vi "Drive and Climb SS Implem 2017.vi"(11 "Robot Commands":T2) -> (3 "Drive Actuator Out":T1={"Left Drive Output"=0.0, "Right Drive Output"=0.0, "Low/High Gear Shift"=enum."Reverse", "Left Climb Shift"=enum."Off", "Right Climb Shift"=enum."Off", "Run Climb Motor"=0.0})   [LabVIEW 2016]
uses:
  Drive + Climb Commands 2017.ctl
  Drive Actuator Out 2017.ctl
  Global Variables/Robot Status.vi
  Global Variables/High Gear Calibrations.vi
  Global Variables/Low Gear Calibrations.vi
  Global Variables/Auto Drive Calibrations.vi
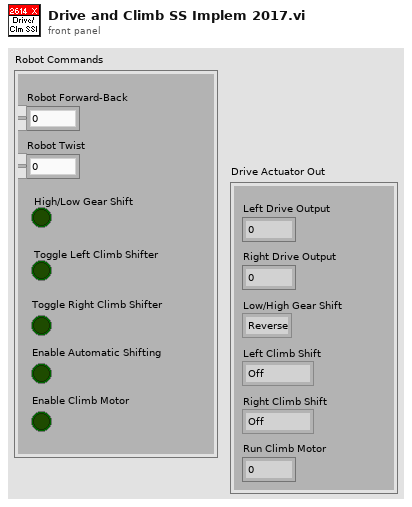
[diagram p1: front panel]
types:
  T1 = typedef "Drive Actuator Out 2017.ctl" = cluster{"Left Drive Output":dbl, "Right Drive Output":dbl, "Low/High Gear Shift":enum16{"Off", "On", "Forward", "Reverse"}, "Left Climb Shift":enum16{"Off", "On", "Forward", "Reverse"}, "Right Climb Shift":enum16{"Off", "On", "Forward", "Reverse"}, "Run Climb Motor":dbl}
  T2 = typedef "Drive + Climb Commands 2017.ctl" = cluster{"Robot Forward-Back":dbl, "Robot Twist":dbl, "High/Low Gear Shift":bool, "Toggle Left Climb Shifter":bool, "Toggle Right Climb Shifter":bool, "Enable Automatic Shifting":bool, "Enable Climb Motor ":bool}
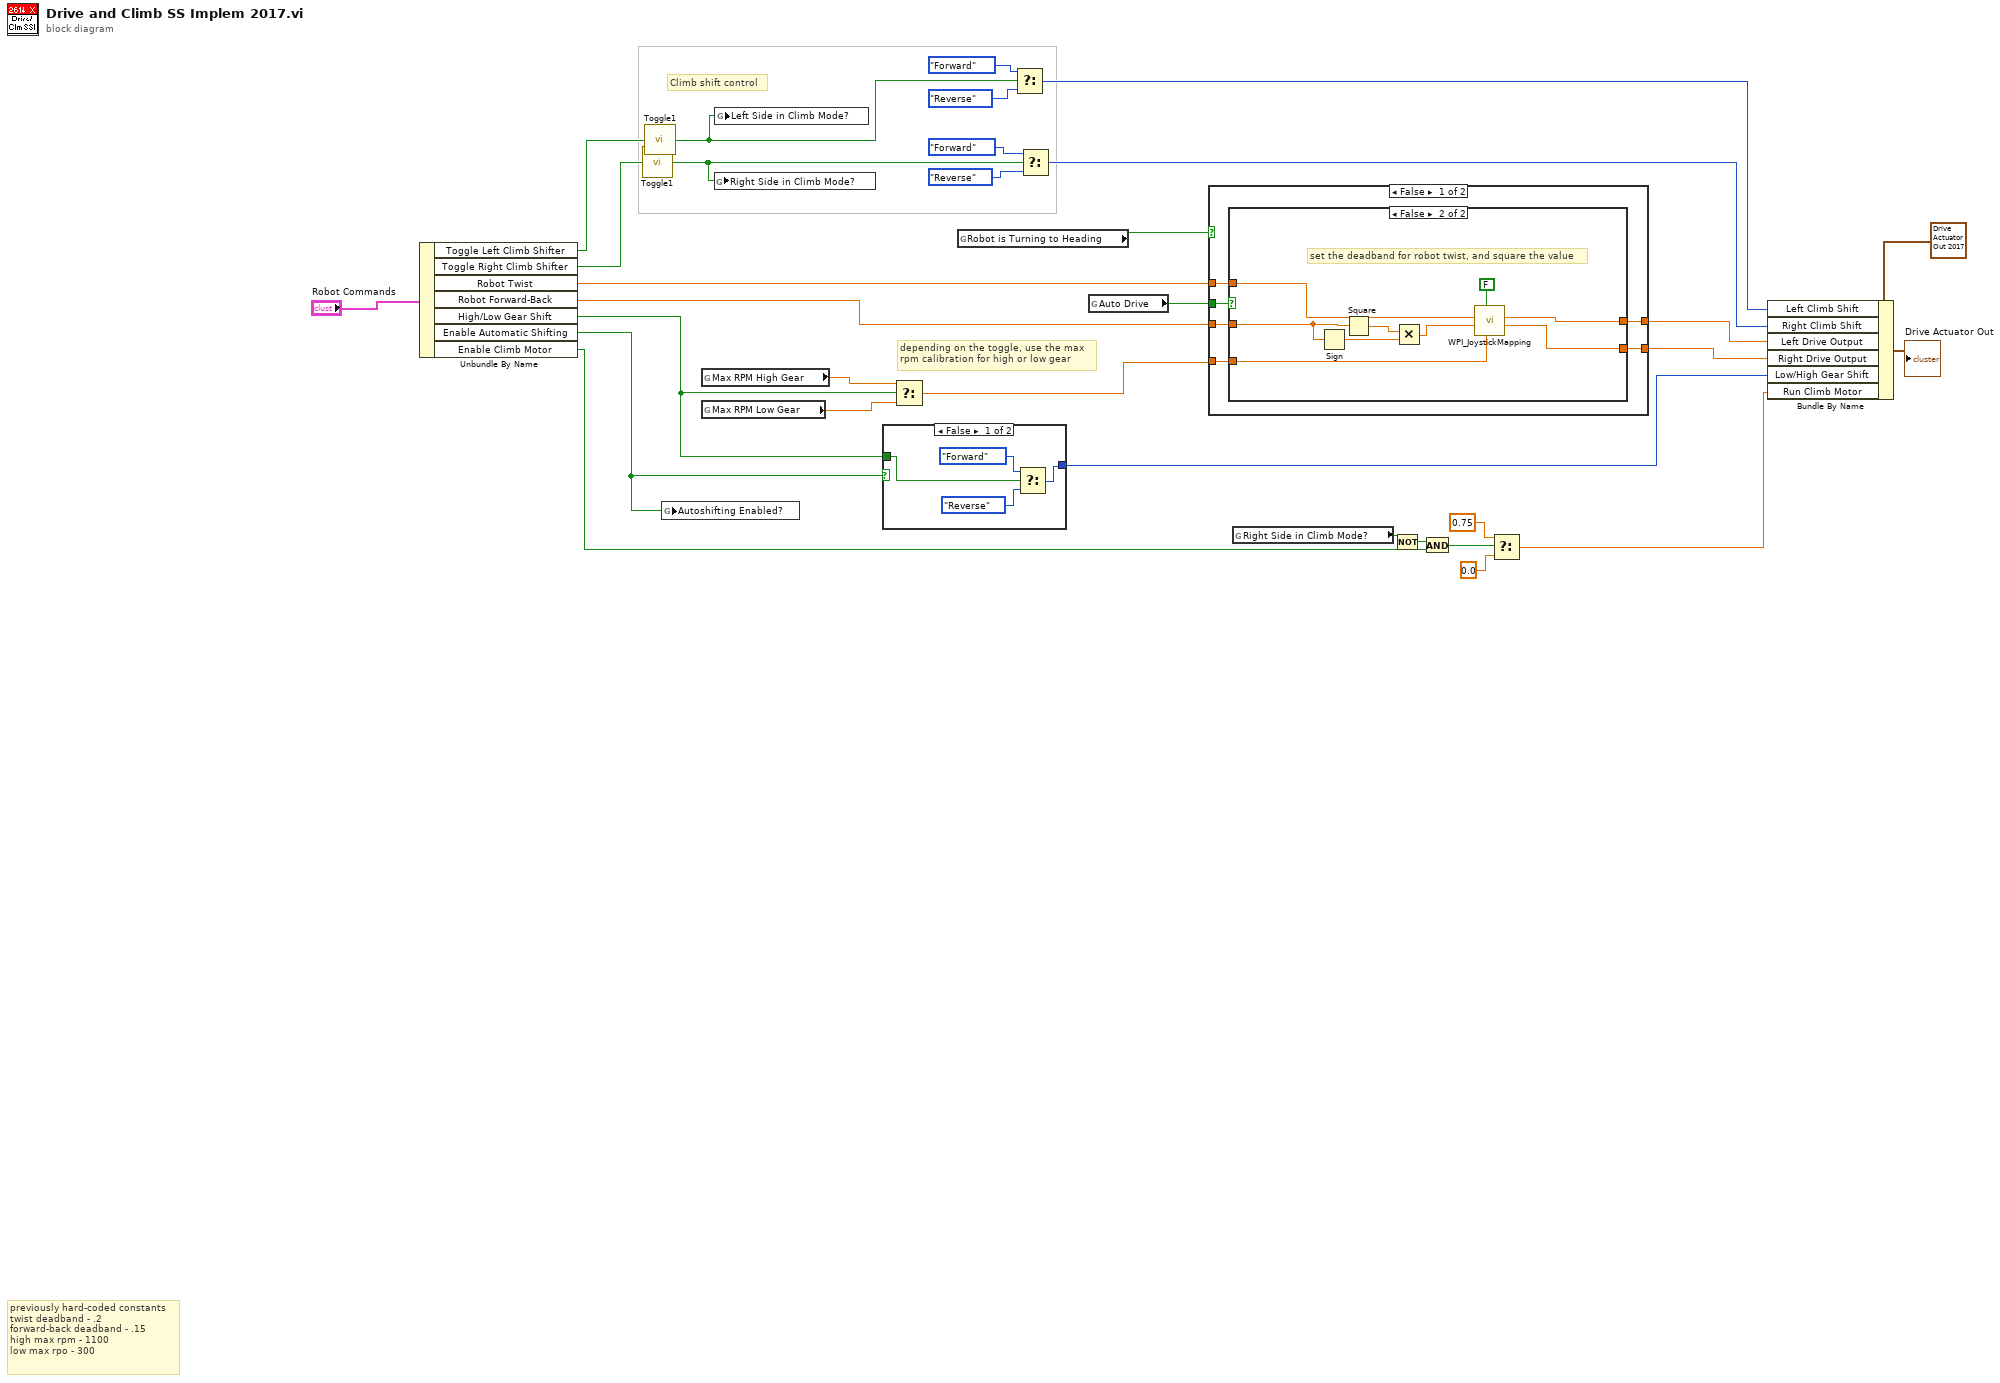
[diagram p0: block diagram]
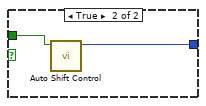
[diagram p2: hidden frame]
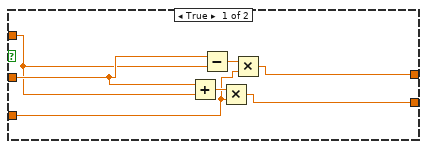
[diagram p3: hidden frame]
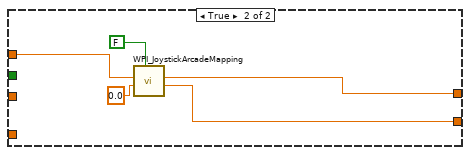
[diagram p4: hidden frame]
diagram:
  # "Climb shift control"
  # "depending on the toggle, use the max\nrpm calibration for high or low gear"
  # "previously hard-coded constants\ntwist deadband - .2\nforward-back deadband - .15\nhigh max rpm - 1100\nlow max rpo - 300"
  n1 = Unbundle By Name("Robot Commands") -> ("Toggle Left Climb Shifter"=w25:bool, "Toggle Right Climb Shifter"=w24:bool, "Robot Twist"=w15:dbl, "Robot Forward-Back"=w10:dbl, "High/Low Gear Shift"=w9:bool, "Enable Automatic Shifting"=w13:bool, "Enable Climb Motor"=w3:bool)
  n2 = call "Toggle1.vi"("Boolean"=w24) -> ("Driver Switch 2"=w16:bool)
  n3 = call "Toggle1.vi"("Boolean"=w25) -> ("Driver Switch 2"=w17:bool)
  n4 = global write "Robot Status.vi" "Autoshifting Enabled?"(w13) -> ()
  n5 = global read "High Gear Calibrations.vi" "Max RPM High Gear"() -> (w26:dbl)
  n6 = global read "Low Gear Calibrations.vi" "Max RPM Low Gear"() -> (w11:dbl)
  n7 = global write "Robot Status.vi" "Right Side in Climb Mode?"(w16) -> ()
  n8 = global write "Robot Status.vi" "Left Side in Climb Mode?"(w17) -> ()
  n9 = case shown="False" w13 {
    tunnel: [w33 w38] -> w12
    tunnel: w9 -> [w35 w37]
    frame False {
      n10 = Select(t=enum16{"Off", "On", "Forward", "Reverse"}."Forward" ("Low/High Gear Shift"), s=w35, f=enum16{"Off", "On", "Forward", "Reverse"}."Reverse" ("Low/High Gear Shift")) -> (s? t:f=w33:enum16{"Off", "On", "Forward", "Reverse"})
    }
    frame True {
      n11 = call "Auto Shift Control.vi"("High/Low Gear Shift"=w37) -> ("Low/High Gear Shift"=w38:enum16{"Off", "On", "Forward", "Reverse"})  [unwired: 10 in]
    }
  }
  n12 = Select(t=w26, s=w9, f=w11) -> (s? t:f=w27:dbl)
  n13 = global read "Robot Status.vi" "Robot is Turning to Heading"() -> (w14:bool)
  n14 = Select(t=enum16{"Off", "On", "Forward", "Reverse"}."Forward" ("Left Climb Shift"), s=w17, f=enum16{"Off", "On", "Forward", "Reverse"}."Reverse" ("Left Climb Shift")) -> (s? t:f=w19:enum16{"Off", "On", "Forward", "Reverse"})
  n15 = Select(t=enum16{"Off", "On", "Forward", "Reverse"}."Forward" ("Left Climb Shift"), s=w16, f=enum16{"Off", "On", "Forward", "Reverse"}."Reverse" ("Left Climb Shift")) -> (s? t:f=w18:enum16{"Off", "On", "Forward", "Reverse"})
  n16 = global read "Auto Drive Calibrations.vi" "Auto Drive"() -> (w8:bool)
  n17 = case shown="False" w14 {
    tunnel: [w42 w63] -> w29
    tunnel: [w43 w62] -> w28
    tunnel: w10 -> [w40 _]
    tunnel: w27 -> [w44 _]
    tunnel: w15 -> [w41 w61]
    tunnel: w8 -> [w39 _]
    frame False {
      n18 = case shown="False" w39 {
        tunnel: w44 -> [w45 w52]
        tunnel: [w50 w59] -> w43
        tunnel: [w51 w58] -> w42
        tunnel: w41 -> [w48 w57]
        tunnel: w40 -> [w49 w56]
        frame True {
          n19 = Add(x=w49, y=w48) -> (x+y=w47:dbl)
          n20 = Subtract(x=w49, y=w48) -> (x-y=w46:dbl)
          n21 = Multiply(x=w47, y=w45) -> (x*y=w50:dbl)
          n22 = Multiply(x=w46, y=w45) -> (x*y=w51:dbl)
        }
        frame False {
          # "set the deadband for robot twist, and square the value"
          n23 = Sign(1:w56) -> (0:w54:dbl)
          n24 = Square(x=w56) -> (x^2=w55:dbl)
          n25 = Multiply(x=w55, y=w54) -> (x*y=w53:dbl)
          n26 = call-poly <vilib>:"WPI_JoystickMapping.vi"("Max Output"=w52, "Square Inputs"=FALSE, "Y axis value"=w53, "X axis value"=w57) -> ("Right Motor Value"=w59:dbl, "Left Motor Value"=w58:dbl)  [unwired: 6 in]
        }
      }
    }
    frame True {
      n27 = call <vilib>:"WPI_JoystickArcadeMapping.vi"("Square Inputs"=FALSE, "Y axis value"=0.0, "X axis value"=w61) -> ("Right Motor Value"=w62:dbl, "Left Motor Value"=w63:dbl)  [unwired: 7 in]
    }
  }
  n28 = global read "Robot Status.vi" "Right Side in Climb Mode?"() -> (w2:bool)
  n29 = Not(x=w2) -> (.not. x?=w1:bool)
  n30 = And(x=w1, y=w3) -> (x .and. y?=w4:bool)
  n31 = Select(t=0.75, s=w4, f=0.0) -> (s? t:f=w7:dbl)
  n32 = Bundle By Name(cluster=T1 {"Left Drive Output"=0.0, "Right Drive Output"=0.0, "Low/High Gear Shift"=enum."Reverse", "Left Climb Shift"=enum."Off", "Right Climb Shift"=enum."Off", "Run Climb Motor"=0.0} ("Drive Actuator Out 2"), "Left Climb Shift"=w19, "Right Climb Shift"=w18, "Left Drive Output"=w29, "Right Drive Output"=w28, "Low/High Gear Shift"=w12, "Run Climb Motor"=w7) -> (→"Drive Actuator Out":T1)
